vi "Tester.vi"() -> ()   [LabVIEW 2020, in "TopModule.lvclass"]
uses:
  TopModule/TopModule.lvclass
  DMM/DMM.lvclass
  C:/Repo/LabVIEW-SOLID-Examples/SOLID-Dataflow-Template/IReference/IRef.lvclass
  VoltageResult/VoltageResult.lvclass
  IAction/IAction.lvclass
  IConfig/IConfig.lvclass
  IResult/IResult.lvclass
  IReference/IRef.lvclass
  VoltageResult/VoltageResult.lvclass/VoltageResult.ctl
  VoltageMeas/VoltageMeas.lvclass
  C:/Repo/LabVIEW-SOLID-Examples/SOLID-Dataflow-Template/IAction/IAction.lvclass
  ConfigA/ConfigA.lvclass
  C:/Repo/LabVIEW-SOLID-Examples/SOLID-Dataflow-Template/IConfig/IConfig.lvclass
  C:/Repo/LabVIEW-SOLID-Examples/SOLID-Dataflow-Template/ConfigA/ConfigA.lvclass
  C:/Repo/LabVIEW-SOLID-Examples/SOLID-Dataflow-Template/DMM/DMM.lvclass
  C:/Repo/LabVIEW-SOLID-Examples/SOLID-Dataflow-Template/VoltageMeas/VoltageMeas.lvclass
panel:
  out "Mean":dbl
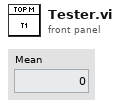
[diagram p1: front panel]
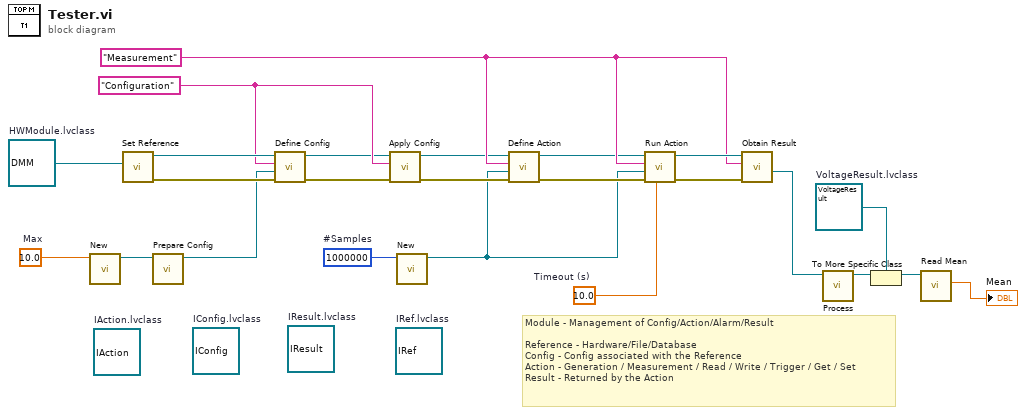
[diagram p0: block diagram]
diagram:
  (unwired) refnum<class "IRef.lvclass"> refnum  # IRef.lvclass
  (unwired) refnum<class "IResult.lvclass"> refnum  # IResult.lvclass
  (unwired) refnum<class "IConfig.lvclass"> refnum  # IConfig.lvclass
  (unwired) refnum<class "IAction.lvclass"> refnum  # IAction.lvclass
  w5 = 10.0  # Max
  w7 = 1000000  # #Samples
  w9 = refnum<class "VoltageResult.lvclass"> refnum  # VoltageResult.lvclass
  w2 = 10.0  # Timeout (s)
  w17 = "Measurement" ("Name")
  w22 = "Configuration" ("Name")
  w24 = refnum<class "DMM.lvclass"> refnum  # HWModule.lvclass
  # "Module - Management of Config/Action/Alarm/Result\n\nReference - Hardware/File/Database\nConfig - Config associated with the Reference\nAction - Generation / Measurement / Read / Write / Trigger / Get / Set\nResult - Returned by the Action"
  n1 = call "New.vi"("Max"=w5) -> ("ConfigA.lvclass"=w6:refnum<class "ConfigA.lvclass">)  [unwired: 10 in]
  n2 = call "Set Reference.vi"("Reference"=w24) -> ("ErrorOut"=w21:errorcluster, "TopModuleOut"=w23:refnum<class "TopModule.lvclass">)  [unwired: 9 in]
  n3 = call "Prepare Config.vi"("IConfig In"=w6) -> ("IConfig Out"=w18:refnum<class "ConfigA.lvclass">)  [unwired: 9 in, 1 out]
  n4 = call "Define Config.vi"("ErrorIn"=w21, "Config"=w18, "Name"=w22, "TopModuleIn"=w23) -> ("ErrorOut"=w15:errorcluster, "TopModuleOut"=w16:refnum<class "TopModule.lvclass">)  [unwired: 6 in]
  n5 = call "Apply Config.vi"("Error In"=w15, "Name"=w22, "TopModule In"=w16) -> ("Error Out"=w13:errorcluster, "TopModule Out"=w14:refnum<class "TopModule.lvclass">)  [unwired: 7 in]
  n6 = call "New.vi"("#Samples"=w7) -> ("VoltageMeas.lvclass"=w1:refnum<class "VoltageMeas.lvclass">)  [unwired: 10 in]
  n7 = call "Define Action.vi"("ErrorIn"=w13, "IAction.lvclass"=w1, "Name"=w17, "TopModuleIn"=w14) -> ("ErrorOut"=w11:errorcluster, "TopModuleOut"=w12:refnum<class "TopModule.lvclass">)  [unwired: 6 in]
  n8 = call "Run Action.vi"("Timeout (s)"=w2, "ErrorIn"=w11, "IAction"=w1, "Action"=w17, "TopModuleIn"=w12) -> ("ErrorOut"=w19:errorcluster, "TopModuleOut"=w20:refnum<class "TopModule.lvclass">)  [unwired: 4 in, 1 out]
  n9 = call "Obtain Result.vi"("ErrorIn"=w19, "Name"=w17, "TopModuleIn"=w20) -> ("ResultOut"=w4:refnum<class "IResult.lvclass">)  [unwired: 5 in, 3 out]
  n10 = call-dynamic "Process.vi"("IResult In"=w4) -> ("IResult Out"=w3:refnum<class "IResult.lvclass">)  [unwired: 9 in, 1 out]
  n11 = To More Specific Class(target class=w9, reference=w3) -> (specific class reference=w10:refnum<class "VoltageResult.lvclass">)  [unwired: 1 in, 1 out]
  n12 = call "Read Mean.vi"("VoltageResultIn"=w10) -> ("Mean"=→"Mean":dbl)  [unwired: 9 in, 1 out]
